vi "Teleop Climb control.vi"(11 "Axes":T1) -> ()   [LabVIEW 2016]
uses:
  Common Code/Gamepads/Axes Cluster.ctl
  Robot Global Data.vi
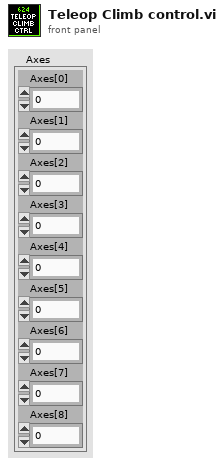
[diagram p1: front panel]
types:
  T1 = typedef "Axes Cluster.ctl" = cluster{"Axes[0]":dbl, "Axes[1]":dbl, "Axes[2]":dbl, "Axes[3]":dbl, "Axes[4]":dbl, "Axes[5]":dbl, "Axes[6]":dbl, "Axes[7]":dbl, "Axes[8]":dbl}
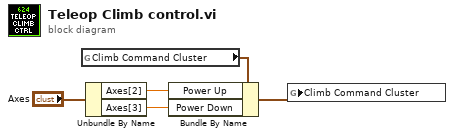
[diagram p0: block diagram]
diagram:
  n1 = global read "Robot Global Data.vi" "Climb Command Cluster"() -> (w4:cluster{"Power Up":dbl, "Power Down":dbl})
  n2 = Unbundle By Name("Axes") -> ("Axes[2]"=w2:dbl, "Axes[3]"=w1:dbl)
  n3 = Bundle By Name(cluster=w4, "Power Up"=w2, "Power Down"=w1) -> (w3:cluster{"Power Up":dbl, "Power Down":dbl})
  n4 = global write "Robot Global Data.vi" "Climb Command Cluster"(w3) -> ()
